vi "TCP Sandbox.vi"() -> ()   [LabVIEW 2019]
panel:
  out "Response":dbl
  in  "Request":string
  in  "Port Number":dbl
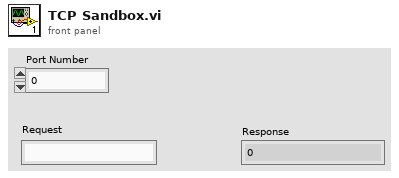
[diagram p1: front panel]
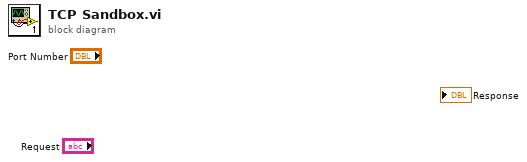
[diagram p0: block diagram]
diagram:
